vi "OkIo.vi"(8 "error in (no error)":errorcluster, 11 "Data In":T2) -> (0 "error out":errorcluster, 1 "States":T1=enum."Initialize", 3 "Data Out":T2)   [LabVIEW 2014]
uses:
  controls/Data1.ctl
  controls/Payjson.ctl
  controls/State.ctl
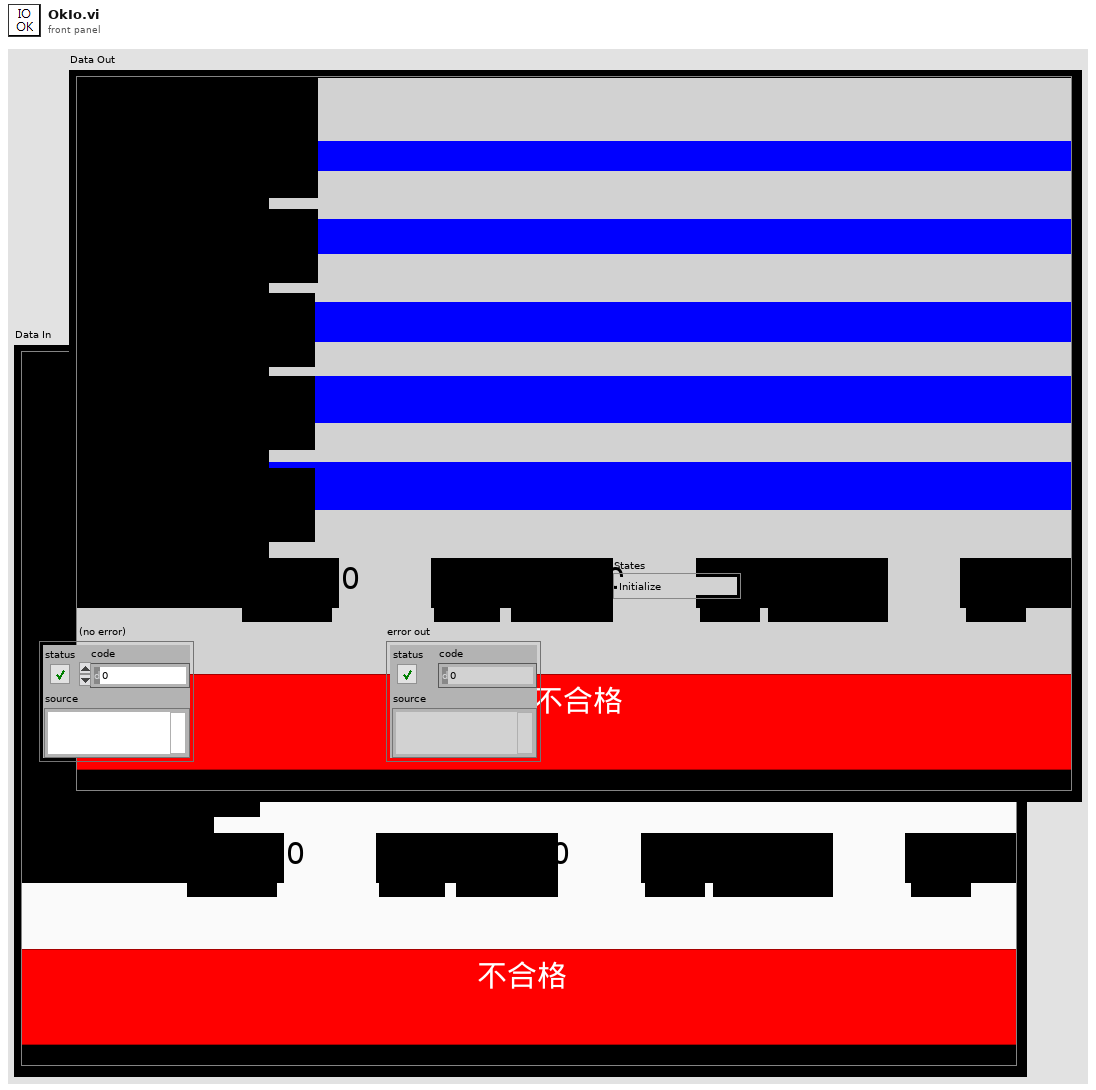
[diagram p1: front panel]
types:
  T1 = typedef "State.ctl" = enum16{"int", "Initalize0", "Initialize", "Wait for Scan", "State 1", "State 2", "NG", "NG1", "OK", "OKNG", "OKNG1", "Exit"}
  T2 = typedef "Data1.ctl" = cluster{"Date":string, "BarCode1":string, "BarCode2":string, "BarCode3":string, "Message":string, "OK Count":u16, "NG Count":u16, "Total Count":u16, "ModelData":string[][], "OK&NG":bool, "COM1":refnum<visa-resource-name>, "COM2":refnum<visa-resource-name>, "IO":i32, "Time":u32, "TCP":refnum<k5>, "TCP 2":refnum<k5>, "COM1 2":refnum<visa-resource-name>, "CheckNum":string, "BarCode1_1":string, "BarCode2_1":string, "BarCode3_1":string, "日期":string, "機種":string, "機號":string, "商品條碼1":string, "OK_1":string, "OK":string, "NG":string, "NG_1":string, "Total":string, "Total_1":string, "ClaerTime":u32, "Pjson":T3, "LotNo":string[], "CheckParsArray":string[], "BarCode4":string, "BarCode4_1":string, "商品條碼2":string, "BarCode5":string, "BarCode5_1":string, "商品條碼3":string, "ReScanNG":i32, "NGTimeCT":u32}
  T3 = typedef "Payjson.ctl" = cluster{"DEPT":string, "LINE":string, "STANO":string, "WORKNO":string, "PRODSN":string, "COMPNTID":string, "COMPNTLOT":string, "COMPNTSN":string, "USEDQTY":i16, "OPDATE":string, "OPUSER":string, "RECVDATE":string, "MMODU":string}[]
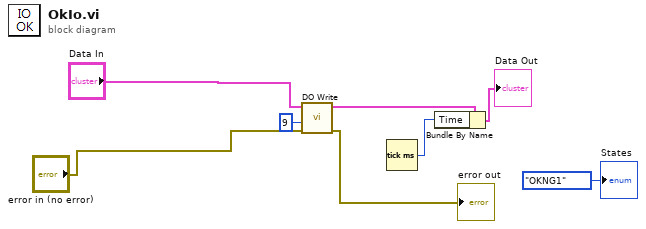
[diagram p0: block diagram]
diagram:
  n1 = call "DO Write.vi"("error in (no error)"="error in (no error)", "data"=u8 9, "Data In"="Data In") -> ("error out"=→"error out":errorcluster, "Data Out"=w3:T2)  [unwired: 7 in]
  n2 = Tick Count (ms)() -> (millisecond timer value=w5:u32)
  n3 = Bundle By Name(cluster=w3, "Time"=w5) -> (→"Data Out":T2)
  "States" <- State."OKNG1" ("States")
